vi "GA_translateDNA.vi"() -> (1 "line_y (500, 20)":dbl[][](array[numeric]), 2 "line_x (500, 20)":dbl[][](array[numeric]))   [LabVIEW 2018]
uses:
  GA_Global.vi
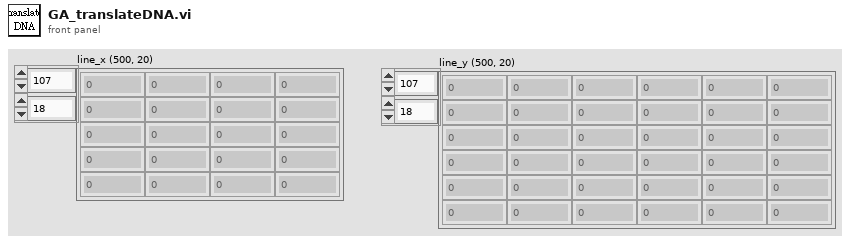
[diagram p1: front panel]
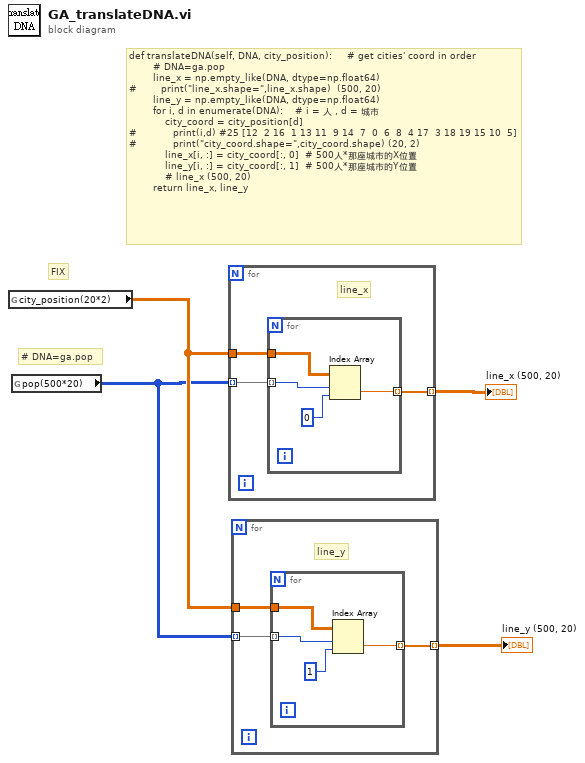
[diagram p0: block diagram]
diagram:
  # "FIX"
  # "# DNA=ga.pop"
  # "def translateDNA(self, DNA, city_position):     # get cities' coord in order\n        # DNA=ga.pop\n        line_x = np.empty_like(DNA, dtype=np.float64) \n#        print(\"line_x.shape=\",line_x.shape)  (500, 20)\n        line_y = np.empty_like(DNA, dtype=np.float64)\n        for i, d in enumerate(DNA):    # i = 人 , d = 城市\n            city_coord = city_position[d]\n#            print(i,d) #25 [12  2 16  1 13 11  9 14  7  0  6  8  4 17  3 18 19 15 10  5]\n#            print(\"city_coord.shape=\",city_coord.shape) (20, 2)\n            line_x[i, :] = city_coord[:, 0]  # 500人*那座城市的X位置\n            line_y[i, :] = city_coord[:, 1]  # 500人*那座城市的Y位置\n            # line_x (500, 20)\n        return line_x, line_y"
  n1 = global read "GA_Global.vi" "city_position(20*2)"() -> (w3:dbl[][])
  n2 = global read "GA_Global.vi" "pop(500*20)"() -> (w2:i32[][])
  n3 = for {
    tunnel: w3 -> [w7]
    tunnel: w2 -> [w6] mode=indexing
    tunnel: [w5] -> w4 mode=indexing
    # "line_x"
    n4 = for {
      tunnel: w7 -> [w11]
      tunnel: w6 -> [w10] mode=indexing
      tunnel: [w8] -> w5 mode=indexing
      n5 = Index Array(array=w11, index (row)=w10, index (col)=0 ("disabled index (col)")) -> (element=w8:dbl)
    }
  }
  "line_x (500, 20)" <- w4
  n6 = for {
    tunnel: w3 -> [w14]
    tunnel: w2 -> [w13] mode=indexing
    tunnel: [w12] -> w1 mode=indexing
    # "line_y"
    n7 = for {
      tunnel: w14 -> [w18]
      tunnel: w13 -> [w17] mode=indexing
      tunnel: [w15] -> w12 mode=indexing
      n8 = Index Array(array=w18, index (row)=w17, index (col)=1 ("disabled index (col)")) -> (element=w15:dbl)
    }
  }
  "line_y (500, 20)" <- w1
